vi "in_Hermite interpolating polynomial.vi"(8 "index i":i32, 9 "Y deriv[0..N]":dbl[](array[numeric]) format="%_6g", 10 "X[0..N]":dbl[](array[numeric]) format="%_6g", 11 "Y[0..N]":dbl[](array[numeric]) format="%_6g") -> (3 "Hermite polynomial":dbl[](array[numeric]) format="%_6g")   [LabVIEW 2013, in "NI_Gmath.lvlib"]
uses:
  NI_Gmath.lvlib
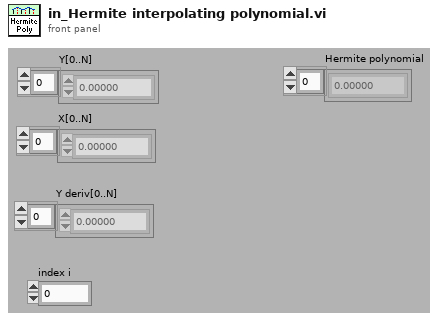
[diagram p1: front panel]
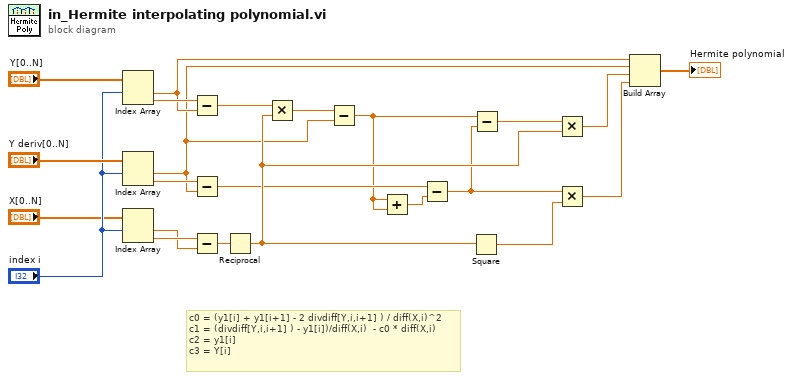
[diagram p0: block diagram]
diagram:
  # "c0 = (y1[i] + y1[i+1] - 2 divdiff[Y,i,i+1] ) / diff(X,i)^2\nc1 = (divdiff[Y,i,i+1] ) - y1[i])/diff(X,i)  - c0 * diff(X,i)\nc2 = y1[i]\nc3 = Y[i]"
  n1 = Index Array(array="Y[0..N]", index #1="index i") -> (element #1=w13:dbl, element #2=w21:dbl)  [unwired: 1 in]
  n2 = Index Array(array="Y deriv[0..N]", index #1="index i") -> (element #1=w3:dbl, element #2=w4:dbl)  [unwired: 1 in]
  n3 = Index Array(array="X[0..N]", index #1="index i") -> (element #1=w16:dbl, element #2=w18:dbl)  [unwired: 1 in]
  n4 = Subtract(x=w21, y=w13) -> (x-y=w20:dbl)
  n5 = Subtract(x=w4, y=w3) -> (x-y=w2:dbl)
  n6 = Subtract(x=w18, y=w16) -> (x-y=w15:dbl)
  n7 = Reciprocal(x=w15) -> (1/x=w9:dbl)
  n8 = Multiply(x=w20, y=w9) -> (x*y=w7:dbl)
  n9 = Subtract(x=w7, y=w3) -> (x-y=w1:dbl)
  n10 = Add(x=w1, y=w1) -> (x+y=w8:dbl)
  n11 = Subtract(x=w2, y=w8) -> (x-y=w6:dbl)
  n12 = Square(x=w9) -> (x^2=w14:dbl)
  n13 = Subtract(x=w1, y=w6) -> (x-y=w5:dbl)
  n14 = Multiply(x=w5, y=w9) -> (x*y=w12:dbl)
  n15 = Multiply(x=w6, y=w14) -> (x*y=w11:dbl)
  n16 = Build Array(w13, w3, w12, w11) -> (→"Hermite polynomial":dbl[])
